vi "setexp.vi"() -> ()   [LabVIEW 2011]
uses:
  Basler - A504 Comm tool.llb/1301_BASLER_A504_TD_commands.ctl
  Basler - A504 Comm tool.llb/M023-01_TDE_Action.ctl
panel:
  out "error out":errorcluster
  in  "Parameter":u32
  out "Ack?":bool
  out "Data":i32
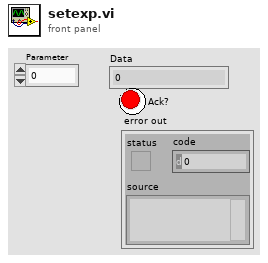
[diagram p1: front panel]
types:
  T1 = typedef "M023-01_TDE_Action.ctl" = enum16{"Read", "Write"}
  T2 = typedef "1301_BASLER_A504_TD_commands.ctl" = enum16{"Read Status", "Exposer Time [us]", "Frame Rate", "ROI start column", "ROI width column", "ROI starting line", "ROI height in lines", "ExSync programmable", "Set Gain", "Set PosOffset", "Set NegOffset", "reset"}
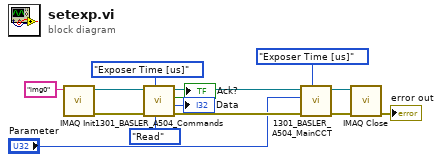
[diagram p0: block diagram]
diagram:
  n1 = call <vilib>:"IMAQ Init.vi"("Interface Name"="img0") -> ("error out"=w10:errorcluster, "IMAQ Session Out"=w8:refnum<k11>)  [unwired: 9 in]
  n2 = call "1301_BASLER_A504_Commands.vi"("Read/Write"=M023-01_TDE_Action."Read", "Commands"=1301_BASLER_A504_TD_commands."Exposer Time [us]", "error in"=w10, "Session In"=w8) -> ("error out"=w9:errorcluster, "Data"=→"Data":i32, "Ack?"=→"Ack?":bool, "Session out"=w7:refnum<k11>)  [unwired: 4 in]
  n3 = call "1301_BASLER_A504_MainCCT.vi"("Commands"=1301_BASLER_A504_TD_commands."Exposer Time [us]", "error in"=w9, "Parameter"="Parameter", "Session In"=w7) -> ("error out"=w1:errorcluster, "Session out"=w2:refnum<k11>)  [unwired: 5 in, 1 out]
  n4 = call <vilib>:"IMAQ Close.vi"("error in (no error)"=w1, "IMAQ Session In"=w2) -> ("error out"=→"error out":errorcluster)  [unwired: 9 in]
